vi "Launch Pane Relief Tool for test.vi"   [LabVIEW 2020]
panel:
  # "RUN THIS VI TO TEST THE PANE RELIEF TOOL"
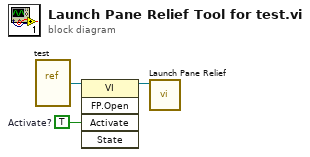
[diagram p0: block diagram]
diagram:
  w1 = TRUE  # Activate?
  n1 = vi-ref "test.vi"() -> (w3:refnum<vi>)
  n2 = invoke class="VI" method="FP.Open"(reference=w3, "Activate"=w1) -> (reference out=w2:refnum<vi>)  [unwired: 3 in, 4 out]
  n3 = call "Launch Pane Relief.vi"("VI in"=w2) -> ()  [unwired: 9 in, 2 out]
